vi "Process.vi"(8 "error in (no error)":errorcluster, 9 "Sensor Groups (false)":bool, 10 "Pound in":refnum<class "Pound.lvclass">, 11 "Qbus in":refnum<class "Qbus.lvclass">) -> (0 "error out":errorcluster)   [LabVIEW 2017, in "ModbusMaster.lvlib"]
uses:
  <vilib>/addons/InsightCM/Devices/Shared/Common/ModbusMaster/ModbusMaster.lvlib
  <vilib>/addons/Qbus/Qbus.lvclass
  <vilib>/NI/Software Watchdog/Pound/Pound.lvclass
  <vilib>/addons/InsightCM/Devices/Shared/Common/ModbusMaster/controls/config.ctl
  <vilib>/addons/InsightCM/Devices/Shared/Common/ModbusMaster/controls/ModbusDevice.ctl
  <vilib>/Modbus/master/Modbus Master.lvclass
  <vilib>/addons/InsightCM/Devices/Shared/Common/ModbusMaster/controls/ModbusChannel.ctl
  <vilib>/addons/InsightCM/Devices/Shared/Common/ModbusMaster/controls/RegisterType.ctl
  <vilib>/addons/InsightCM/MessageBus/Base/controls/DataSource.ctl
  <vilib>/addons/InsightCM/MessageBus/Base/controls/KeyValuePair.ctl
  <vilib>/NI/Software Watchdog/Watchdog/Watchdog.lvclass
  <vilib>/addons/TraceLogger/TraceLogger.lvlib
  <vilib>/addons/InsightCM/Utilities/GlobalConfiguration/GlobalConfiguration.lvlib
  <vilib>/addons/InsightCM/Utilities/PropertyHelpers/PropertyHelpers.lvlib
  <vilib>/addons/InsightCM/Devices/Shared/Common/ServerComm/ServerComm.lvlib
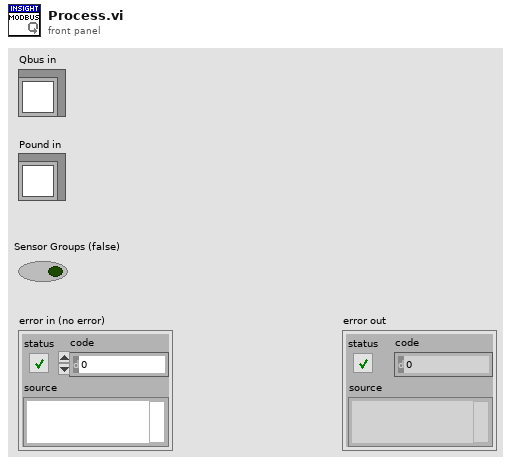
[diagram p1: front panel]
types:
  T1 = typedef "ModbusMaster.lvlib/config.ctl" = cluster{"Devices":T2[], "ReadTimeout":i32}
  T2 = typedef "ModbusMaster.lvlib/ModbusDevice.ctl" = cluster{"reference":refnum<class "Modbus Master.lvclass">, "Serial":bool, "ReadInterval (sec)":dbl, "ReadTimeout (ms)":i32, "LastRead":dbl, "channels":T3[], "connected":bool, "DataSource":T5}
  T3 = typedef "ModbusMaster.lvlib/ModbusChannel.ctl" = cluster{"RegisterType":T4, "Address":i32, "32bitRegister":bool, "FirstWordLow":bool, "FloatingPoint":bool, "Slope":dbl, "Offset":dbl, "ValueTag":string, "Name":string, "Range Check":bool, "MinimumEU":dbl, "MaximumEU":dbl, "Groups":string[]}
  T4 = typedef "ModbusMaster.lvlib/RegisterType.ctl" = enum16{"Unknown", "Coil", "Discrete Input", "Holding Register", "Input Register"}
  T5 = typedef "DataSource.ctl" = cluster{"Id":string, "Type":string, "Name":string, "MeasType":string, "Properties":T6[]}
  T6 = typedef "KeyValuePair.ctl" = cluster{"Key":string, "Value":string}
  T7 = typedef "SectionKeyValues.ctl" = cluster{"Section":string, "KeyValues":T6[]}
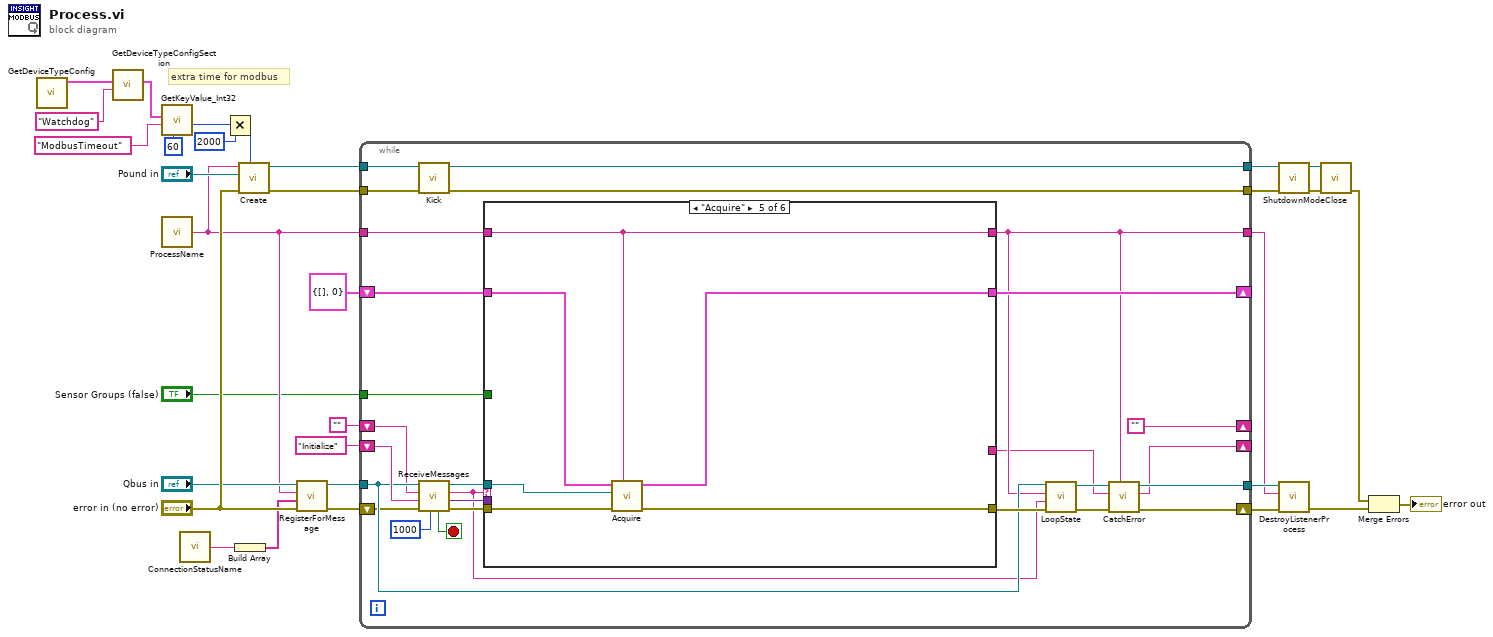
[diagram p0: block diagram]
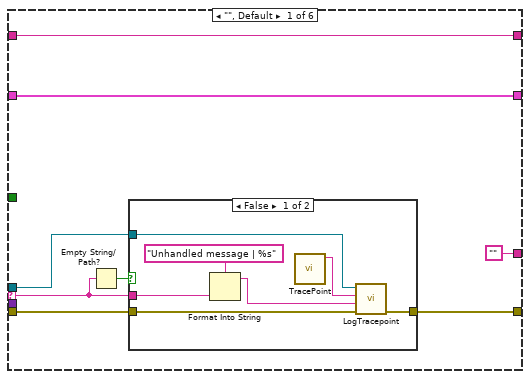
[diagram p2: hidden frame]
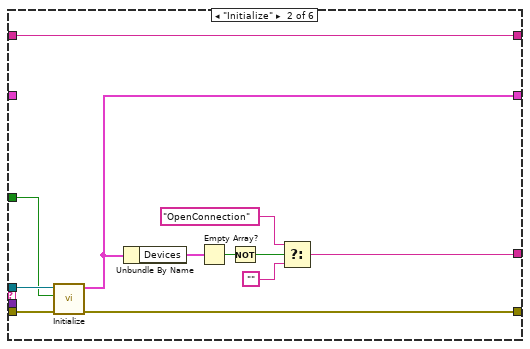
[diagram p4: hidden frame]
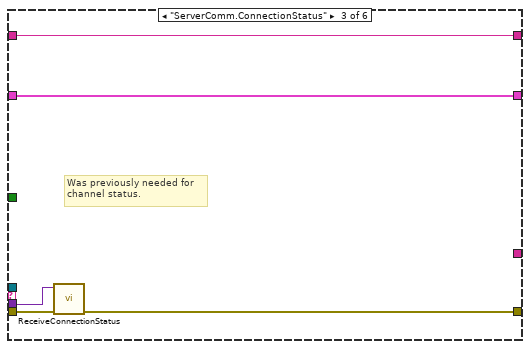
[diagram p5: hidden frame]
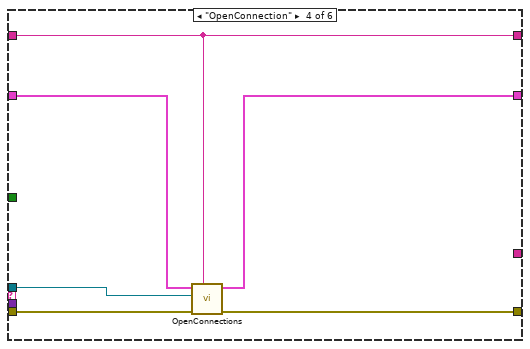
[diagram p6: hidden frame]
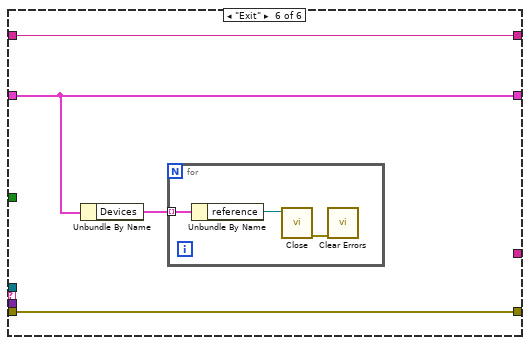
[diagram p7: hidden frame]
diagram:
  # "extra time for modbus"
  n1 = call <vilib>:"GetDeviceTypeConfig.vi"() -> ("key values"=w16:T7[])  [unwired: 9 in, 2 out]
  n2 = call <vilib>:"GetDeviceTypeConfigSection.vi"("key"="Watchdog", "key values"=w16) -> ("key value pairs out"=w13:T6[])  [unwired: 8 in, 1 out]
  n3 = call <vilib>:"GetKeyValue_Int32.vi"("default"=60, "key"="ModbusTimeout" ("Tag"), "key value pairs"=w13) -> ("value"=w10:i32)  [unwired: 6 in, 2 out]
  n4 = call <vilib>:"ProcessName.vi"() -> ("process name"=w4:string)  [unwired: 5 in]
  n5 = call <vilib>:"ConnectionStatusName.vi"() -> ("message name"=w3:string)  [unwired: 5 in]
  n6 = Multiply(x=w10, y=2000) -> (x*y=w9:i32)
  n7 = Build Array(w3) -> (w2:string[])
  n8 = call <vilib>:"Create.vi"("Execution Timeout (ms)"=w9, "error in (no error)"="error in (no error)", "Pound"="Pound in", "Name"=w4) -> ("error out"=w21:errorcluster, "Watchdog"=w26:refnum<data-value>)  [unwired: 6 in]
  n9 = call <vilib>:"RegisterForMessage.vi"("error in (no error)"="error in (no error)", "message names"=w2, "process name"=w4, "Qbus in"="Qbus in") -> ("error in (no error)"=w7:errorcluster, "Qbus out"=w5:refnum<class "Qbus.lvclass">)  [unwired: 6 in]
  n10 = while {
    shift-right: [""] -> _
    shift-left: "" -> [w35]
    tunnel: w5 -> [w48]
    tunnel: w4 -> [w38]
    tunnel: [w51] -> w30
    tunnel: [w37] -> w29
    shift-right: [w50] -> _
    shift-left: "Initialize" -> [w55]
    shift-right: [w53] -> _
    shift-left: T1 {"Devices"=[], "ReadTimeout"=0} ("config") -> [w54]
    tunnel: w26 -> [w47]
    tunnel: [w46] -> w23
    tunnel: w21 -> [w45]
    tunnel: [w43] -> w20
    shift-right: [w52] -> w31
    shift-left: w7 -> [w44]
    tunnel: "Sensor Groups (false)" -> [w33]
    stop <- w59 stop-if-true
    n11 = call <vilib>:"Kick.vi"("error in (no error)"=w45, "Watchdog"=w47) -> ("error out"=w43:errorcluster, "Watchdog"=w46:refnum<data-value>)  [unwired: 8 in]
    n12 = call <vilib>:"ReceiveMessages.vi"("Timeout(1000)"=1000 ("milliseconds to wait"), "error in (no error)"=w44, "priority action"=w55, "default action"=w35, "Qbus in"=w48) -> ("error out"=w58:errorcluster, "message value"=w56:variant, "action"=w42:string, "Qbus out"=w57:refnum<class "Qbus.lvclass">, "exit"=w59:bool)  [unwired: 2 in]
    n13 = case shown="\"Acquire\"" w42 {
      selector: w42 -> [w63 _ _ _ _ _]
      tunnel: w58 -> [w65 w85 w91 w98 w104 w108]
      tunnel: w57 -> [w61 w86 _ w95 w100 _]
      tunnel: [w64 w84 w90 w94 w101 w108] -> w49
      tunnel: w56 -> [_ _ w89 _ _ _]
      tunnel: w54 -> [w67 _ w88 w97 w103 w106]
      tunnel: [w67 w80 w88 w96 w102 w106] -> w53
      tunnel: [w66 w87 w92 w93 w99 w107] -> w37
      tunnel: w38 -> [w66 w87 w92 w93 w99 w107]
      tunnel: ["" w81 _ _ _ _] -> w36
      tunnel: w33 -> [_ w76 _ _ _ _]
      frame "", Default {
        n14 = Empty String/Path?(string/path=w63) -> (empty?=w62:bool)
        n15 = case shown="False" w62 {
          tunnel: [w71 w75] -> w64
          tunnel: w65 -> [w72 w75]
          tunnel: w63 -> [w74 _]
          tunnel: w61 -> [w70 _]
          frame False {
            n16 = Format Into String(format string="Unhandled message | %s", w74) -> (resulting string=w69:string)  [unwired: 2 in, 1 out]
            n17 = call <vilib>:"TracePoint.vi"() -> ("template trace point"=w68:string)  [unwired: 11 in]
            n18 = call <vilib>:"LogTracepoint.vi"("error in (no error)"=w72, "log string"=w69, "tracepoint"=w68, "qbus in"=w70) -> ("error out"=w71:errorcluster)  [unwired: 6 in, 1 out]
          }
          frame True {
          }
        }
      }
      frame "Initialize" {
        n19 = call <vilib>:"Initialize.vi"("error in (no error)"=w85, "Sensor Groups (false)"=w76, "Qbus"=w86) -> ("error out"=w84:errorcluster, "config"=w80:T1)  [unwired: 7 in]
        n20 = Unbundle By Name(w80) -> ("Devices"=w79:T2[])
        n21 = Empty Array?(array=w79) -> (empty?=w78:bool)
        n22 = Not(x=w78) -> (.not. x?=w77:bool)
        n23 = Select(t="OpenConnection", s=w77, f="") -> (s? t:f=w81:string)
      }
      frame "ServerComm.ConnectionStatus" {
        # "Was previously needed for\nchannel status."
        n24 = call <vilib>:"ReceiveConnectionStatus.vi"("error in (no error)"=w91, "body"=w89) -> ("error out"=w90:errorcluster)  [unwired: 6 in, 3 out]
      }
      frame "OpenConnection" {
        n25 = call <vilib>:"OpenConnections.vi"("process name"=w93, "error in (no error)"=w98, "Qbus"=w95, "config in"=w97) -> ("error out"=w94:errorcluster, "config out"=w96:T1)  [unwired: 6 in]
      }
      frame "Acquire" {
        n26 = call <vilib>:"Acquire.vi"("process name"=w99, "error in (no error)"=w104, "Qbus in"=w100, "config in"=w103) -> ("error out"=w101:errorcluster, "config out"=w102:T1)  [unwired: 6 in]
      }
      frame "Exit" {
        n27 = Unbundle By Name(w106) -> ("Devices"=w105:T2[])
        n28 = for {
          tunnel: w105 -> [w111] mode=indexing
          n29 = Unbundle By Name(w111) -> ("reference"=w110:refnum<class "Modbus Master.lvclass">)
          n30 = call-dynamic <vilib>:"Close.vi"("Modbus master in"=w110) -> ("error out"=w109:errorcluster)  [unwired: 10 in]
          n31 = call <vilib>:"Clear Errors.vi"("error in (no error)"=w109) -> ()  [unwired: 5 in, 2 out]
        }
      }
    }
    n32 = call <vilib>:"LoopState.vi"("error in (no error)"=w49, "loop action"=w42, "process name"=w37, "Qbus in"=w48) -> ("error out"=w40:errorcluster, "Qbus out"=w39:refnum<class "Qbus.lvclass">)  [unwired: 6 in]
    n33 = call <vilib>:"CatchError.vi"("source"=w37, "error in (no error)"=w40, "next action in"=w36, "Qbus in"=w39) -> ("error out"=w52:errorcluster, "next action out"=w50:string, "Qbus out"=w51:refnum<class "Qbus.lvclass">)  [unwired: 5 in]
  }
  n34 = call <vilib>:"ShutdownMode.vi"("error in (no error)"=w20, "Watchdog"=w23) -> ("error out"=w22:errorcluster, "Watchdog"=w24:refnum<data-value>)  [unwired: 8 in]
  n35 = call <vilib>:"DestroyListenerProcess.vi"("error in (no error)"=w31, "process name"=w29, "Qbus in"=w30) -> ("error in (no error)"=w19:errorcluster)  [unwired: 7 in, 1 out]
  n36 = call <vilib>:"Close.vi"("error in (no error)"=w22, "Watchdog"=w24) -> ("error out"=w18:errorcluster)  [unwired: 9 in]
  n37 = Merge Errors(w18, w19) -> (→"error out":errorcluster)
